vi "Loop test.vi"() -> ()   [LabVIEW 2017]
panel:
  in  "Start":dbl format="%#_13g"
  in  "End":dbl
  in  "Increment":dbl
  out "Array":dbl[](array[numeric])
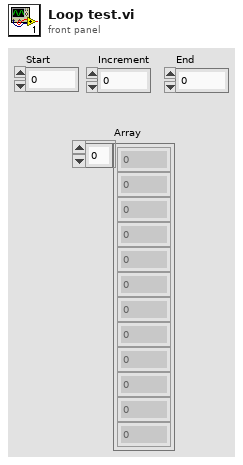
[diagram p1: front panel]
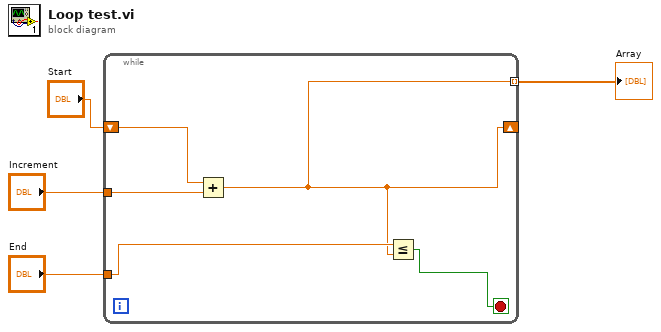
[diagram p0: block diagram]
diagram:
  n1 = while {
    tunnel: [w6] -> w3 mode=indexing
    shift-right: [w6] -> _
    shift-left: "Start" -> [w8]
    tunnel: "Increment" -> [w9]
    tunnel: "End" -> [w7]
    stop <- w5 stop-if-true
    n2 = Add(x=w8, y=w9) -> (x+y=w6:dbl)
    n3 = Less Or Equal?(x=w7, y=w6) -> (x <= y?=w5:bool)
  }
  "Array" <- w3
